vi "add_freq_char_to_report.vi"(8 "error in (no error)":errorcluster, 11 "Boc6 in":refnum<class "Boc6.lvclass">) -> (0 "error out":errorcluster, 3 "Boc6 out":refnum<class "Boc6.lvclass">)   [LabVIEW 2017, in "Boc6.lvclass"]
uses:
  Boc6.lvclass
  Report.lvclass
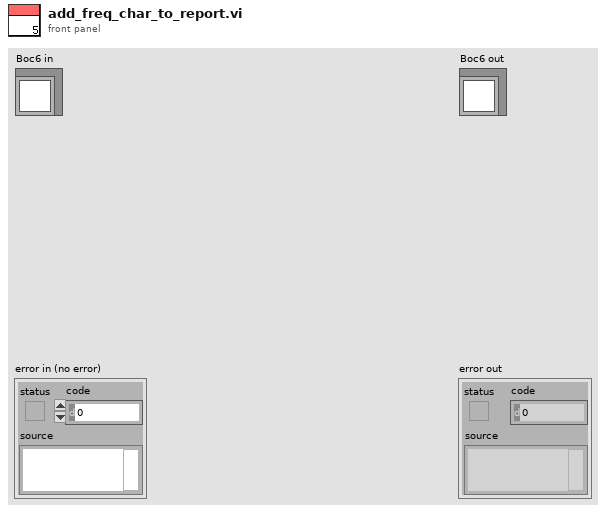
[diagram p1: front panel]
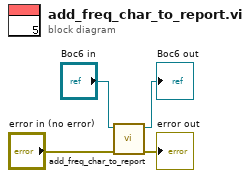
[diagram p0: block diagram]
diagram:
  n1 = call-parent "add_freq_char_to_report.vi"("error in (no error)"="error in (no error)", "Report in"="Boc6 in") -> ("error out"=→"error out":errorcluster, "Report out"=→"Boc6 out":refnum<class "Boc6.lvclass">)  [unwired: 8 in]
